vi "pp_sessList_load.vi"(8 "error in (no error)":errorcluster) -> (0 "error out":errorcluster, 2 "Session List (Cannot Edit)":i32[](array[numeric]), 3 "Session List File Path":path)   [LabVIEW 2013]
uses:
  <vilib>/Utility/file.llb/Read From Spreadsheet File (I64).vi
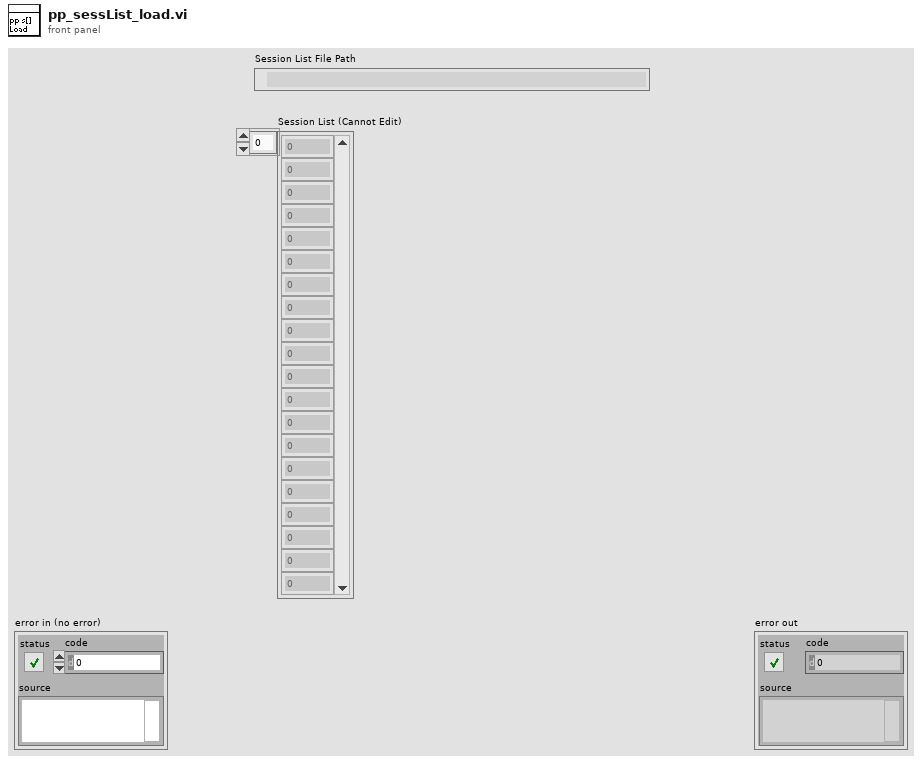
[diagram p1: front panel]
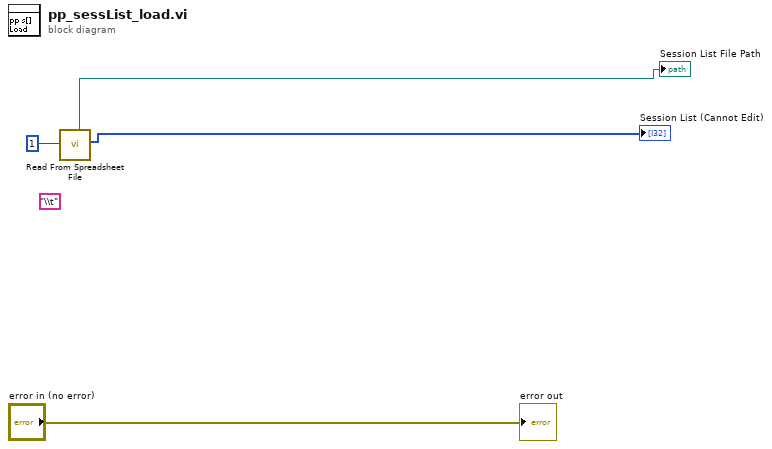
[diagram p0: block diagram]
diagram:
  (unwired) "\\t" ("delimiter (\\t)")
  n1 = call-poly <vilib>:"Read From Spreadsheet File.vi"("number of rows (all:-1)"=1) -> ("first row"=→"Session List (Cannot Edit)":i64[], "new file path (Not A Path if cancelled)"=→"Session List File Path":path)  [unwired: 6 in, 3 out]
  "error out" <- "error in (no error)"
